vi "ConvertFloatToString.vi"(11 "thickness average":dbl) -> (3 "String":string)   [LabVIEW 2013]
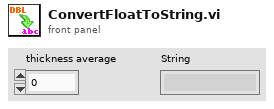
[diagram p1: front panel]
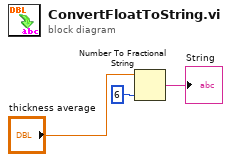
[diagram p0: block diagram]
diagram:
  n1 = Number To Fractional String(number="thickness average", precision (6)=i16 6) -> (F-format string=→"String":string)  [unwired: 2 in]
